vi "Start CPU Calculation.vi"(8 "error in (no error)":errorcluster, 11 "Application Manager in":refnum<class "Application Manager.lvclass">) -> (0 "error out":errorcluster, 3 "Application Manager out":refnum<class "Application Manager.lvclass">)   [LabVIEW 2020, in "Application Manager.lvlib" / "Application Manager.lvclass"]
uses:
  Application Manager.lvclass
  Application Manager.lvclass/Application Manager.ctl
  <vilib>/ActorFramework/Message Enqueuer/Message Enqueuer.lvclass/Message Enqueuer.ctl
  <vilib>/ActorFramework/Message Enqueuer/Enqueue.vi
  CPU FFT Calculator/CPU FFT Calculator Messages/Start Calculation Msg/Start Calculation Msg.lvclass
  C:/Program Files/National Instruments/LabVIEW 2026/vi.lib/ActorFramework/Message/Message.lvclass
  <vilib>/ActorFramework/Message Priority Queue/Priority Enqueue.vi
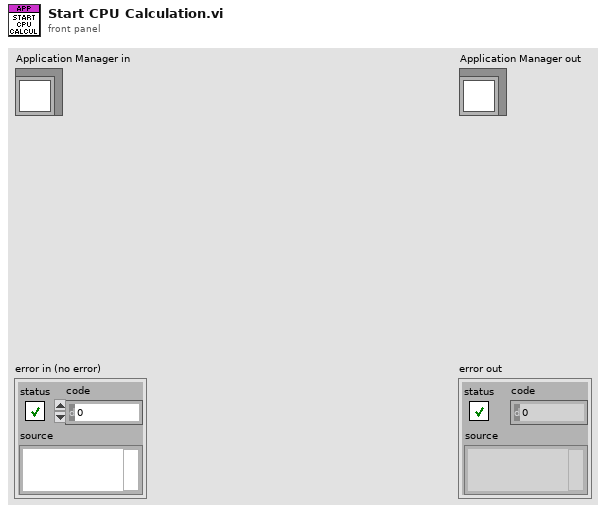
[diagram p1: front panel]
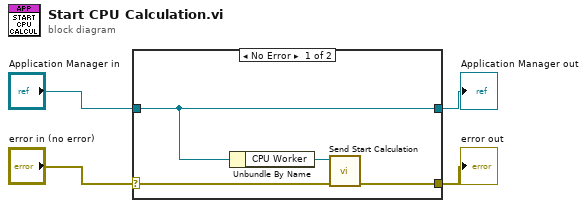
[diagram p0: block diagram]
diagram:
  n1 = case shown="No Error" "error in (no error)" {
    selector: "error in (no error)" -> [w8 w10]
    tunnel: [w7 w10] -> w3
    tunnel: [w6 w9] -> w1
    tunnel: "Application Manager in" -> [w6 w9]
    frame No Error {
      n2 = Unbundle By Name(w6) -> ("CPU Worker"=w5:refnum<class "Message Enqueuer.lvclass">)
      n3 = call "Send Start Calculation.vi"("error in (no error)"=w8, "Message Enqueuer"=w5) -> ("error out"=w7:errorcluster)  [unwired: 8 in, 1 out]
    }
    frame Error {
    }
  }
  "error out" <- w3
  "Application Manager out" <- w1
